vi "Parse ID From Answer.vi"(8 "error in (no error)":errorcluster, 11 "JSON":string) -> (0 "error out":errorcluster, 1 "id-string empty?":bool, 3 "id-string":string, 5 "JSON-input found":bool)   [LabVIEW 2023, in "Communicator.lvclass"]
uses:
  Communicator.lvclass
  <vilib>/JDP Science/JSONtext/Next JSON Value.vi
  <vilib>/JDP Science/JSONtext/String Subset.vi
  <vilib>/JDP Science/JSONtext/Parsing/Advance past next JSON Value (inlined COPY).vi
  <vilib>/JDP Science/JSONtext/Parsing/Advance past whitespace.vi
  <vilib>/JDP Science/JSONtext/Parsing/Advance past String.vi
  <vilib>/JDP Science/JSONtext/Parsing/Advance past Number.vi
  <vilib>/JDP Science/JSONtext/Parsing/Advance past Line Ending.vi
  <vilib>/JDP Science/JSONtext/Parsing/Parse Full Path or Item Name.vi
  <vilib>/JDP Science/JSONtext/Parsing/Advance past Array.vi
  <vilib>/JDP Science/JSONtext/Parsing/Advance past Object.vi
  <vilib>/JDP Science/JSONtext/support/Error Cluster From Code.vi
  <vilib>/JDP Science/JSONtext/Offset/Find Item Locations by Path.vi
  Communicator.lvclass/Communicator.ctl
  <vilib>/JDP Science/JSONtext/JSONtext.lvlib
panel:
  # "Connector Pane"
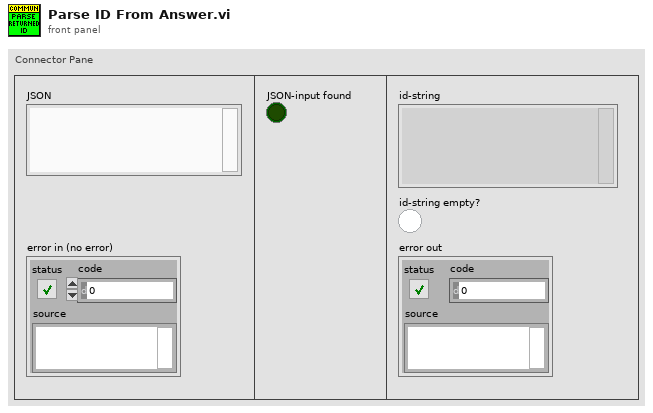
[diagram p1: front panel]
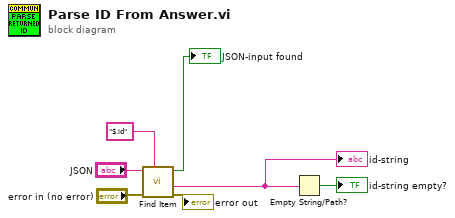
[diagram p0: block diagram]
diagram:
  n1 = call <vilib>:"Find Item.vi"("$Path or Item Name"="$.id", "error in (no error)"="error in (no error)", "JSON"="JSON") -> ("error out"=→"error out":errorcluster, "<JSON>"=w2:string, "Found"=→"JSON-input found":bool)  [unwired: 5 in, 1 out]
  "id-string" <- w2
  n2 = Empty String/Path?(string/path=w2) -> (empty?=→"id-string empty?":bool)
